vi "dlltest_int8.vi"() -> ()   [LabVIEW 2020]
uses:
  source/repos/cont2019/x64/Release/Image_processing.dll
panel:
  out "maxium":u8
  out "Intensity Graph":i8[][](graph)
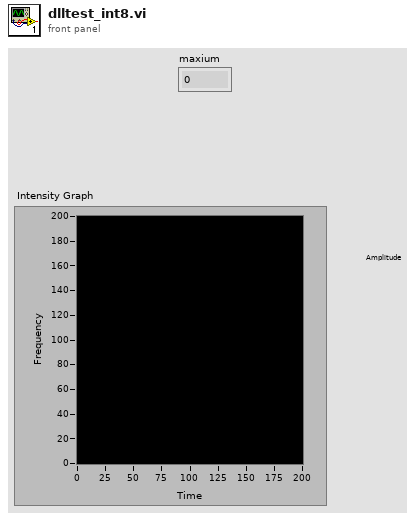
[diagram p1: front panel]
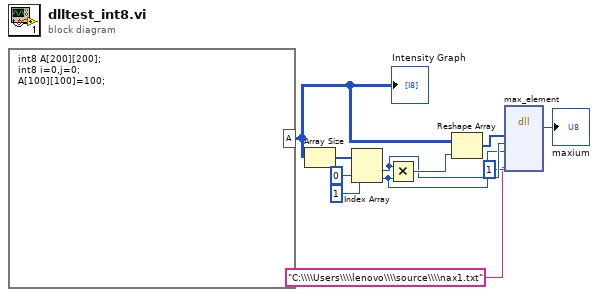
[diagram p0: block diagram]
diagram:
  n1 = formula code="int8 A[200][200];\nint8 i=0,j=0;\nA[100][100]=100;"() -> ("A"=w11:i8[][])
  "Intensity Graph" <- w11
  n2 = Array Size(array=w11) -> (size(s)=w10:i32[])
  n3 = Index Array(array=w10, index #1=0 ("index"), index #2=1 ("index")) -> (element #1=w5:i32, element #2=w4:i32)
  n4 = Multiply(x=w5, y=w4) -> (x*y=w7:i32)
  n5 = Reshape Array(w11, w7) -> (w6:i8[])
  n6 = dll-call lib="C:/Users/lenovo/source/repos/cont2019/x64/Release/Image_processing.dll" fn="max_element"("pixel_data"=w6, "width"=w5, "height"=w4, "log_data"=1, "path"="C:\\\\Users\\\\lenovo\\\\source\\\\nax1.txt") -> ("maxium"=→"maxium":u8)  [unwired: 8 in, 2 out]
